vi "例6.3 以电子表格格式存储和读取数据.vi"() -> ()   [LabVIEW 2017]
uses:
  <vilib>/Utility/file.llb/Write Delimited Spreadsheet (DBL).vi
  <vilib>/Utility/file.llb/Read Delimited Spreadsheet (DBL).vi
panel:
  out "all rows":dbl[][](array[numeric]) caption="所有行" format="%0.3f"
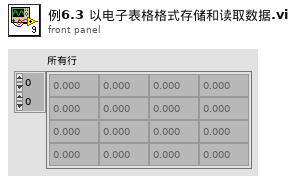
[diagram p1: front panel]
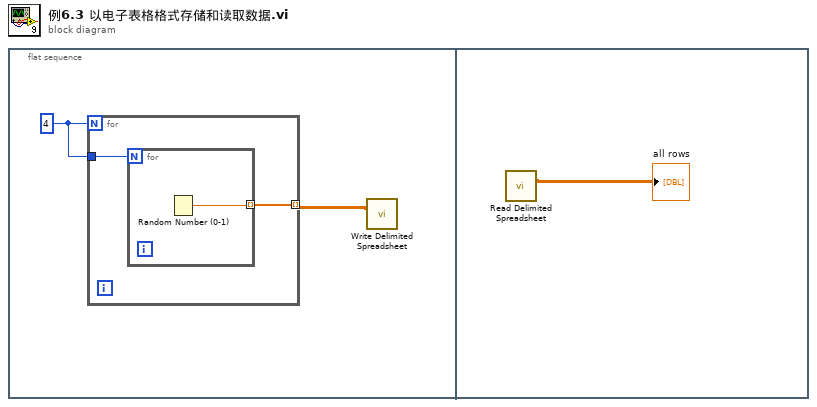
[diagram p0: block diagram]
diagram:
  n1 = flat-sequence {
    frame #0 {
      w2 = 4
      n2 = for {
        N: w2 -> [_]
        tunnel: w2 -> [w4]
        tunnel: [w3] -> w1 mode=indexing
        n3 = for {
          N: w4 -> [_]
          tunnel: [w5] -> w3 mode=indexing
          n4 = Random Number (0-1)() -> (number: 0 to 1=w5:dbl)
        }
      }
      n5 = call-poly <vilib>:"Write Delimited Spreadsheet.vi"("2D data"=w1) -> ()  [unwired: 13 in, 2 out]
    }
    frame #1 {
      n6 = call-poly <vilib>:"Read Delimited Spreadsheet.vi"() -> ("all rows"=→"all rows":dbl[][])  [unwired: 10 in, 5 out]
    }
  }
